vi "2025_day2.vi"() -> ()   [LabVIEW 2025]
panel:
  out "Task 2":u64
  out "Task 1":u64
  in  "Switch":bool caption="Ex. Data  vs.  User Data"
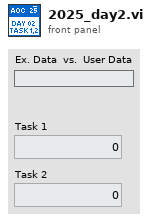
[diagram p1: front panel]
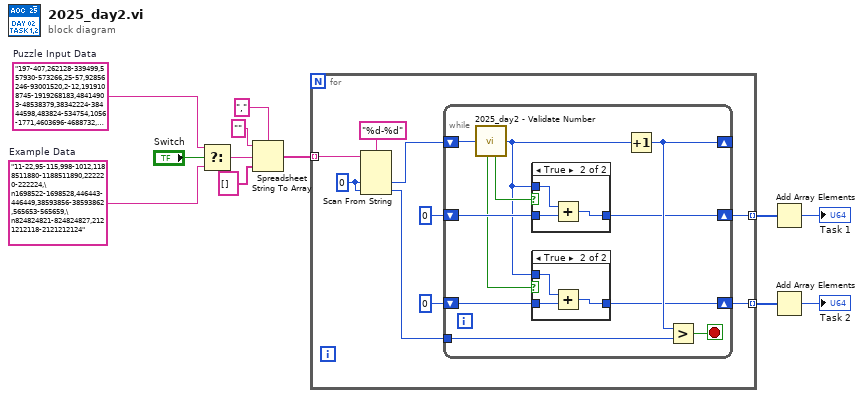
[diagram p0: block diagram]
diagram:
  w10 = "197-407,262128-339499,557930-573266,25-57,92856246-93001520,2-12,1919108745-1919268183,48414903-48538379,38342224-38444598,483824-534754,1056-1771,4603696-4688732,75712519-75792205,20124-44038,714164-782292,4429019-4570680,9648251-9913729,6812551522-6812585188,58-134,881574-897488,648613-673853,5261723647-5261785283,60035-128980,9944818-10047126,857821365-857927915,206885-246173,1922-9652,424942-446151,408-1000"  # Puzzle Input Data
  w11 = "11-22,95-115,998-1012,1188511880-1188511890,222220-222224,\n1698522-1698528,446443-446449,38593856-38593862,565653-565659,\n824824821-824824827,2121212118-2121212124"  # Example Data
  n1 = Select(t=w10, s="Switch", f=w11) -> (s? t:f=w8:string)
  n2 = Spreadsheet String To Array(delimiter (Tab)=",", format string="", spreadsheet string=w8, array type (2D Dbl)=string[] [] ("array")) -> (array=w5:string[])
  n3 = for {
    tunnel: w5 -> [w20] mode=indexing
    tunnel: [w15] -> w4 mode=indexing
    tunnel: [w14] -> w1 mode=indexing
    w17 = u64 0 ("default value 14")
    n4 = Scan From String(format string="%d-%d", input string=w20, default 1=w17, default 2=w17) -> (output 1=w19:u64, output 2=w18:u64)  [unwired: 2 in, 3 out]
    n5 = while {
      shift-right: [w29] -> _
      shift-left: w19 -> [w30]
      tunnel: w18 -> [w31]
      shift-right: [w27] -> w15
      shift-left: u64 0 ("default value 14") -> [w28]
      shift-right: [w25] -> w14
      shift-left: u64 0 ("default value 14") -> [w24]
      stop <- w32 stop-if-true
      n6 = call "2025_day2 - Validate Number.vi"("Number to test In"=w30) -> ("Reptetive Pattern Found? (Task 2)"=w23:bool, "Number to test Out"=w22:u64, "Reptetive Pattern Found? (Task 1)"=w26:bool)  [unwired: 6 in]
      n7 = case shown="True" w26 {
        tunnel: w28 -> [w37 w40]
        tunnel: [w37 w39] -> w27
        tunnel: w22 -> [_ w38]
        frame False {
        }
        frame True {
          n8 = Add(x=w38, y=w40) -> (x+y=w39:u64)
        }
      }
      n9 = case shown="True" w23 {
        tunnel: w24 -> [w33 w36]
        tunnel: [w33 w35] -> w25
        tunnel: w22 -> [_ w34]
        frame False {
        }
        frame True {
          n10 = Add(x=w34, y=w36) -> (x+y=w35:u64)
        }
      }
      n11 = Increment(x=w22) -> (x+1=w29:u64)
      n12 = Greater?(x=w29, y=w31) -> (0:w32:bool)
    }
  }
  n13 = Add Array Elements(numeric array=w4) -> (sum=→"Task 1":u64)
  n14 = Add Array Elements(numeric array=w1) -> (sum=→"Task 2":u64)
